vi "Launcher.vi"   [LabVIEW 2024]
uses:
  Root Actor/Root Actor.lvclass
  Kitchen Actor/Kitchen Actor.lvclass
  <vilib>/ActorFramework/Actor/Actor.lvclass
  C:/Program Files/National Instruments/LabVIEW 2024/vi.lib/ActorFramework/Actor/Actor.lvclass
  C:/Users/burakkorkmaz/Desktop/Leveling/repo/Kitchen Actor/Kitchen Actor.lvclass
  C:/Users/burakkorkmaz/Desktop/Leveling/repo/Kitchen Messaging Interface/Kitchen Messaging Interface/Kitchen Messaging Interface.lvclass
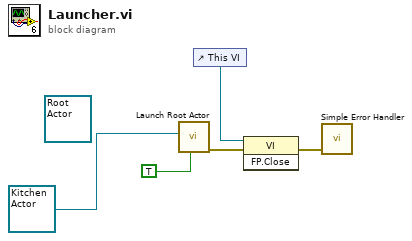
[diagram p0: block diagram]
diagram:
  (unwired) refnum<class "Root Actor.lvclass"> refnum ("Root Actor.lvlib:Root Actor.lvclass")
  n1 = call <vilib>:"Launch Root Actor.vi"("Open Actor Core front panel? (F)"=TRUE, "Actor"=refnum<class "Kitchen Actor.lvclass"> refnum ("Kitchen Actor.lvlib:Kitchen Actor.lvclass")) -> ("error out"=w4:errorcluster)  [unwired: 8 in, 1 out]
  n2 = control-ref of="This VI"() -> (w5:refnum<vi>)
  n3 = invoke class="VI" method="FP.Close"(reference=w5, error in=w4) -> (error out=w3:errorcluster)  [unwired: 1 in, 2 out]
  n4 = call <vilib>:"Simple Error Handler.vi"("error in (no error)"=w3) -> ()  [unwired: 4 in, 5 out]
